vi "Configure Math.vi"(0 "VISA resource name":refnum<visa-resource-name>, 1 "Analysis Range (X) (0: Band Marker X)":u16(ring) items=["Band Marker X", "Full Range"], 5 "Measurement Type (6: Phase Noise)":u16(ring)=6 items=["AM Noise"=1, "Baseband Noise"=2, "Freq/Power"=3, "Spectrum"=4, "Transient"=5, "Phase Noise"=6, "User"=7], 7 "Select Trace (1: 1)":u16(ring)=1 items=["1"=1, "2"=2, "3"=3, "4"=4, "5"=5, "6"=6, "7"=7, "8"=8], 9 "Trace Offset (0)":dbl format="%^#_9g", 11 "error in (no error)":errorcluster, 12 "Analysis Range (Y) (0: Band Marker Y)":u16(ring) items=["Band Marker Y", "Full Range"]) -> (4 "VISA resource name out":refnum<visa-resource-name>, 15 "error out":errorcluster)   [LabVIEW 2011, in "Agilent E5052X.lvlib"]
doc: "Configures the instrument for math functions to be applied to measurements."
uses:
  Agilent E5052X.lvlib
panel:
  # "Analysis Range Settings"
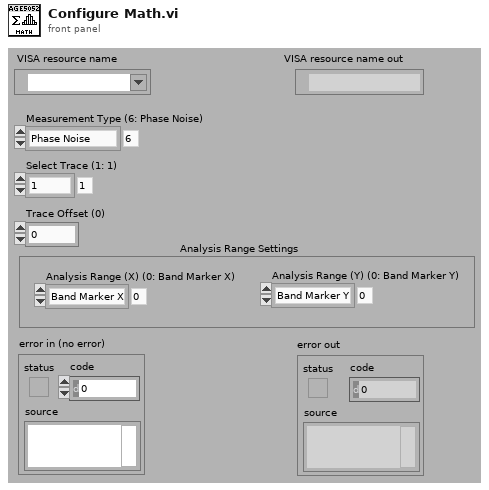
[diagram p1: front panel]
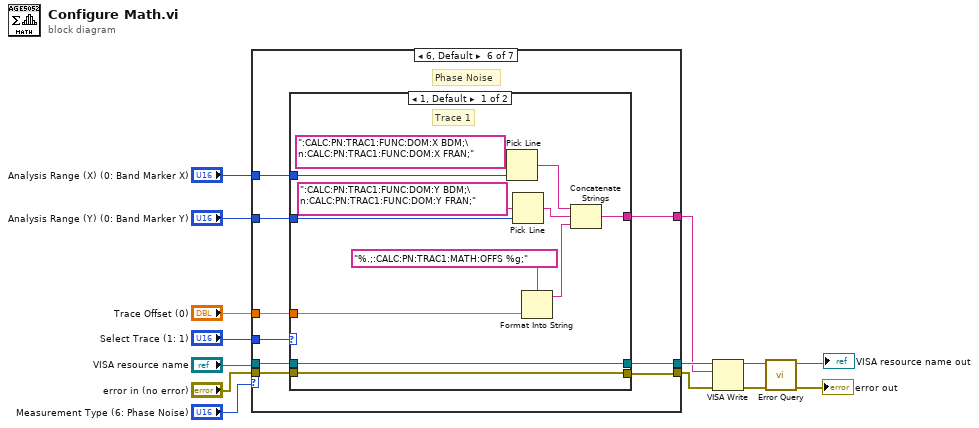
[diagram p0: block diagram]
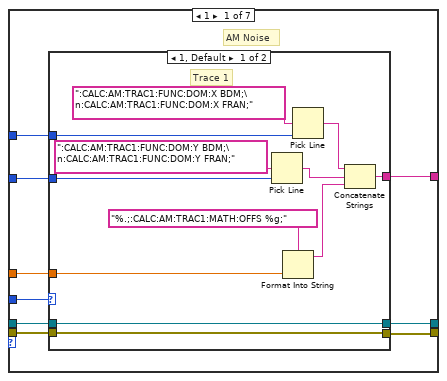
[diagram p2: hidden frame]
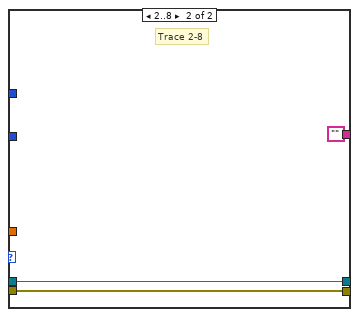
[diagram p3: hidden frame]
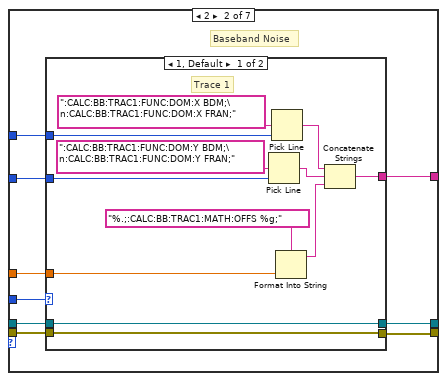
[diagram p4: hidden frame]
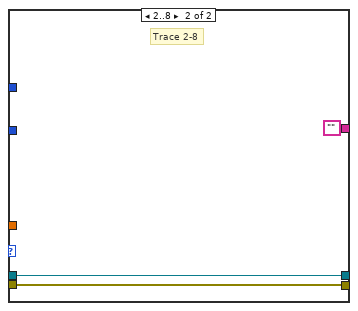
[diagram p5: hidden frame]
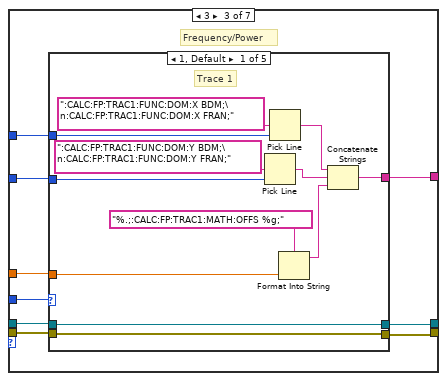
[diagram p6: hidden frame]
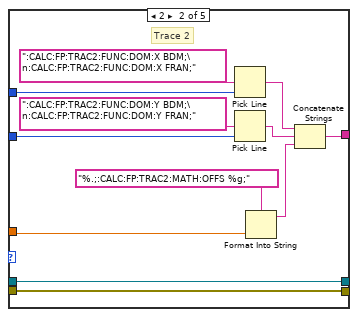
[diagram p7: hidden frame]
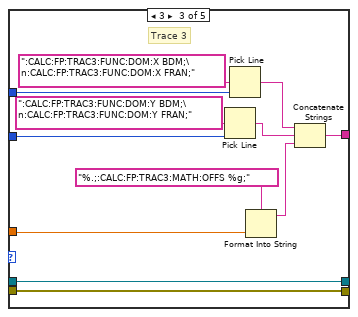
[diagram p8: hidden frame]
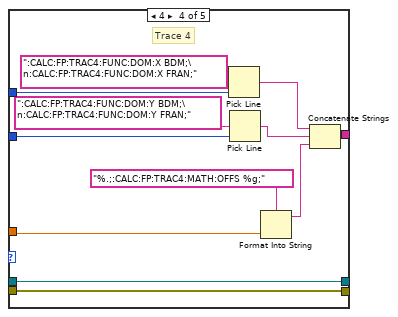
[diagram p9: hidden frame]
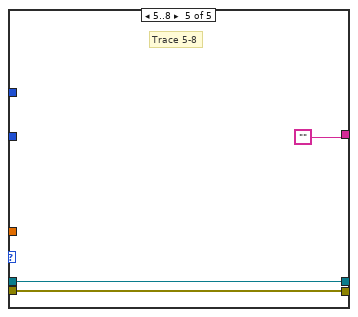
[diagram p10: hidden frame]
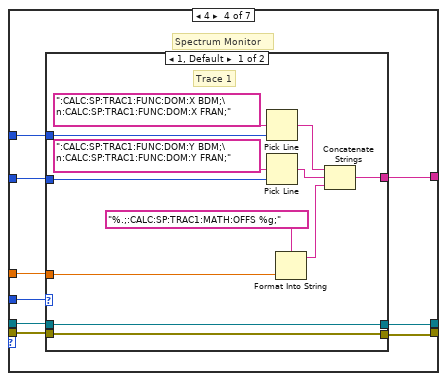
[diagram p11: hidden frame]
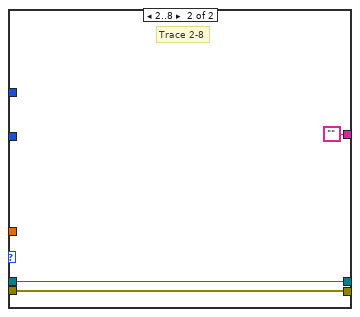
[diagram p12: hidden frame]
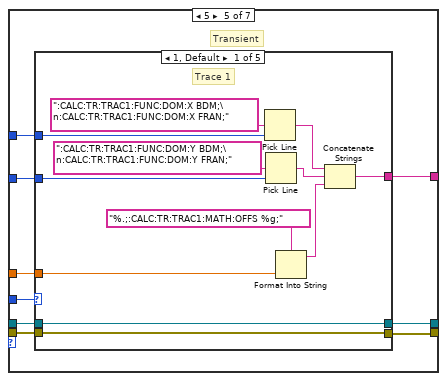
[diagram p13: hidden frame]
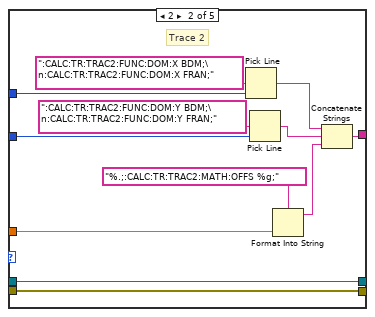
[diagram p14: hidden frame]
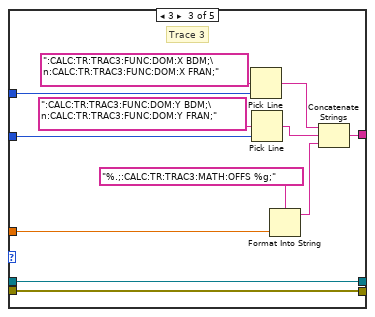
[diagram p15: hidden frame]
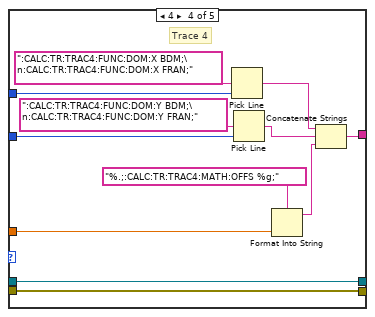
[diagram p16: hidden frame]
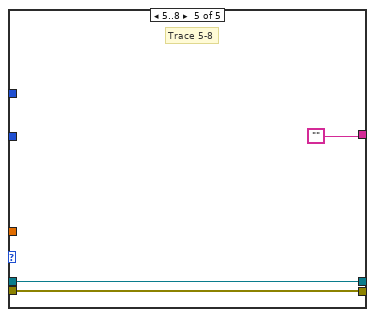
[diagram p17: hidden frame]
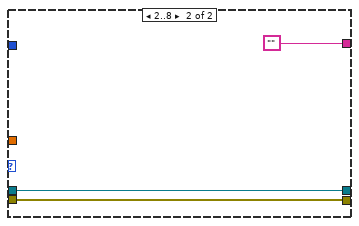
[diagram p18: hidden frame]
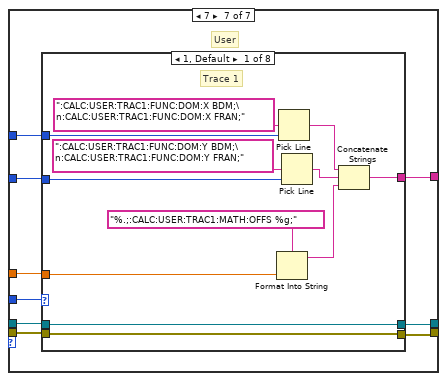
[diagram p19: hidden frame]
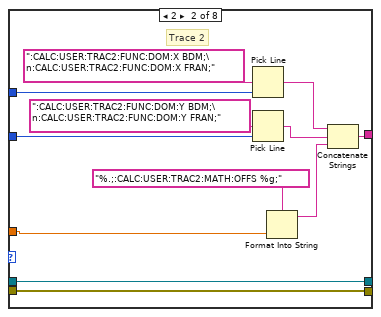
[diagram p20: hidden frame]
diagram:
  n1 = case shown="6, Default" "Measurement Type (6: Phase Noise)" {
    tunnel: "VISA resource name" -> [w23 w44 w68 w127 w151 w211 w235]
    tunnel: "error in (no error)" -> [w22 w43 w67 w126 w150 w210 w234]
    tunnel: "Select Trace (1: 1)" -> [w21 w39 w63 w128 w152 w212 w238]
    tunnel: "Trace Offset (0)" -> [w20 w45 w69 w129 w153 w213 w239]
    tunnel: "Analysis Range (Y) (0: Band Marker Y)" -> [w19 w46 w70 w130 w154 w214 w236]
    tunnel: "Analysis Range (X) (0: Band Marker X)" -> [w18 w47 w71 w131 w155 w215 w237]
    tunnel: [w17 w42 w64 w125 w149 w209 w231] -> w9
    tunnel: [w16 w41 w66 w124 w148 w208 w233] -> w11
    tunnel: [w15 w40 w65 w123 w147 w207 w232] -> w10
    frame 1 {
      # "AM Noise"
      n2 = case shown="1, Default" w21 {
        tunnel: w23 -> [w31 w38]
        tunnel: w22 -> [w30 w37]
        tunnel: w20 -> [w34 _]
        tunnel: w19 -> [w25 _]
        tunnel: w18 -> [w28 _]
        tunnel: [w32 ""] -> w17
        tunnel: [w31 w38] -> w16
        tunnel: [w30 w37] -> w15
        frame 1, Default {
          # "Trace 1"
          n3 = Pick Line(multi-line string=":CALC:AM:TRAC1:FUNC:DOM:Y BDM;\n:CALC:AM:TRAC1:FUNC:DOM:Y FRAN;", line index=w25) -> (output string=w24:string)  [unwired: 1 in]
          n4 = Format Into String(format string="%.;:CALC:AM:TRAC1:MATH:OFFS %g;", w34) -> (resulting string=w33:string)  [unwired: 2 in, 1 out]
          n5 = Pick Line(multi-line string=":CALC:AM:TRAC1:FUNC:DOM:X BDM;\n:CALC:AM:TRAC1:FUNC:DOM:X FRAN;", line index=w28) -> (output string=w27:string)  [unwired: 1 in]
          n6 = Concatenate Strings(w27, w24, w33) -> (w32:string)
        }
        frame 2..8 {
          # "Trace 2-8"
        }
      }
    }
    frame 2 {
      # "Baseband Noise"
      n7 = case shown="1, Default" w39 {
        tunnel: w44 -> [w55 w62]
        tunnel: w43 -> [w54 w61]
        tunnel: w45 -> [w58 _]
        tunnel: w46 -> [w49 _]
        tunnel: w47 -> [w52 _]
        tunnel: [w56 ""] -> w42
        tunnel: [w55 w62] -> w41
        tunnel: [w54 w61] -> w40
        frame 1, Default {
          # "Trace 1"
          n8 = Pick Line(multi-line string=":CALC:BB:TRAC1:FUNC:DOM:Y BDM;\n:CALC:BB:TRAC1:FUNC:DOM:Y FRAN;", line index=w49) -> (output string=w48:string)  [unwired: 1 in]
          n9 = Pick Line(multi-line string=":CALC:BB:TRAC1:FUNC:DOM:X BDM;\n:CALC:BB:TRAC1:FUNC:DOM:X FRAN;", line index=w52) -> (output string=w51:string)  [unwired: 1 in]
          n10 = Format Into String(format string="%.;:CALC:BB:TRAC1:MATH:OFFS %g;", w58) -> (resulting string=w57:string)  [unwired: 2 in, 1 out]
          n11 = Concatenate Strings(w51, w48, w57) -> (w56:string)
        }
        frame 2..8 {
          # "Trace 2-8"
        }
      }
    }
    frame 3 {
      # "Frequency/Power"
      n12 = case shown="1, Default" w63 {
        tunnel: w68 -> [w79 w95 w107 w119 w121]
        tunnel: w67 -> [w78 w94 w106 w118 w120]
        tunnel: w69 -> [w82 w91 w103 w115 _]
        tunnel: w70 -> [w73 w85 w97 w109 _]
        tunnel: w71 -> [w76 w88 w101 w112 _]
        tunnel: [w80 w90 w102 w114 ""] -> w64
        tunnel: [w79 w95 w107 w119 w121] -> w66
        tunnel: [w78 w94 w106 w118 w120] -> w65
        frame 1, Default {
          # "Trace 1"
          n13 = Pick Line(multi-line string=":CALC:FP:TRAC1:FUNC:DOM:Y BDM;\n:CALC:FP:TRAC1:FUNC:DOM:Y FRAN;", line index=w73) -> (output string=w72:string)  [unwired: 1 in]
          n14 = Pick Line(multi-line string=":CALC:FP:TRAC1:FUNC:DOM:X BDM;\n:CALC:FP:TRAC1:FUNC:DOM:X FRAN;", line index=w76) -> (output string=w75:string)  [unwired: 1 in]
          n15 = Format Into String(format string="%.;:CALC:FP:TRAC1:MATH:OFFS %g;", w82) -> (resulting string=w81:string)  [unwired: 2 in, 1 out]
          n16 = Concatenate Strings(w75, w72, w81) -> (w80:string)
        }
        frame 2 {
          # "Trace 2"
          n17 = Pick Line(multi-line string=":CALC:FP:TRAC2:FUNC:DOM:X BDM;\n:CALC:FP:TRAC2:FUNC:DOM:X FRAN;", line index=w88) -> (output string=w87:string)  [unwired: 1 in]
          n18 = Pick Line(multi-line string=":CALC:FP:TRAC2:FUNC:DOM:Y BDM;\n:CALC:FP:TRAC2:FUNC:DOM:Y FRAN;", line index=w85) -> (output string=w84:string)  [unwired: 1 in]
          n19 = Format Into String(format string="%.;:CALC:FP:TRAC2:MATH:OFFS %g;", w91) -> (resulting string=w92:string)  [unwired: 2 in, 1 out]
          n20 = Concatenate Strings(w87, w84, w92) -> (w90:string)
        }
        frame 3 {
          # "Trace 3"
          n21 = Pick Line(multi-line string=":CALC:FP:TRAC3:FUNC:DOM:Y BDM;\n:CALC:FP:TRAC3:FUNC:DOM:Y FRAN;", line index=w97) -> (output string=w96:string)  [unwired: 1 in]
          n22 = Pick Line(multi-line string=":CALC:FP:TRAC3:FUNC:DOM:X BDM;\n:CALC:FP:TRAC3:FUNC:DOM:X FRAN;", line index=w101) -> (output string=w100:string)  [unwired: 1 in]
          n23 = Format Into String(format string="%.;:CALC:FP:TRAC3:MATH:OFFS %g;", w103) -> (resulting string=w104:string)  [unwired: 2 in, 1 out]
          n24 = Concatenate Strings(w100, w96, w104) -> (w102:string)
        }
        frame 4 {
          # "Trace 4"
          n25 = Pick Line(multi-line string=":CALC:FP:TRAC4:FUNC:DOM:X BDM;\n:CALC:FP:TRAC4:FUNC:DOM:X FRAN;", line index=w112) -> (output string=w111:string)  [unwired: 1 in]
          n26 = Pick Line(multi-line string=":CALC:FP:TRAC4:FUNC:DOM:Y BDM;\n:CALC:FP:TRAC4:FUNC:DOM:Y FRAN;", line index=w109) -> (output string=w108:string)  [unwired: 1 in]
          n27 = Format Into String(format string="%.;:CALC:FP:TRAC4:MATH:OFFS %g;", w115) -> (resulting string=w116:string)  [unwired: 2 in, 1 out]
          n28 = Concatenate Strings(w111, w108, w116) -> (w114:string)
        }
        frame 5..8 {
          # "Trace 5-8"
        }
      }
    }
    frame 4 {
      # "Spectrum Monitor"
      n29 = case shown="1, Default" w128 {
        tunnel: w127 -> [w139 w146]
        tunnel: w126 -> [w138 w145]
        tunnel: w129 -> [w142 _]
        tunnel: w130 -> [w133 _]
        tunnel: w131 -> [w136 _]
        tunnel: [w140 ""] -> w125
        tunnel: [w139 w146] -> w124
        tunnel: [w138 w145] -> w123
        frame 1, Default {
          # "Trace 1"
          n30 = Pick Line(multi-line string=":CALC:SP:TRAC1:FUNC:DOM:X BDM;\n:CALC:SP:TRAC1:FUNC:DOM:X FRAN;", line index=w136) -> (output string=w135:string)  [unwired: 1 in]
          n31 = Pick Line(multi-line string=":CALC:SP:TRAC1:FUNC:DOM:Y BDM;\n:CALC:SP:TRAC1:FUNC:DOM:Y FRAN;", line index=w133) -> (output string=w132:string)  [unwired: 1 in]
          n32 = Format Into String(format string="%.;:CALC:SP:TRAC1:MATH:OFFS %g;", w142) -> (resulting string=w141:string)  [unwired: 2 in, 1 out]
          n33 = Concatenate Strings(w135, w132, w141) -> (w140:string)
        }
        frame 2..8 {
          # "Trace 2-8"
        }
      }
    }
    frame 5 {
      # "Transient"
      n34 = case shown="1, Default" w152 {
        tunnel: w151 -> [w163 w179 w191 w203 w205]
        tunnel: w150 -> [w162 w178 w190 w202 w204]
        tunnel: w153 -> [w166 w175 w187 w199 _]
        tunnel: w154 -> [w157 w169 w181 w194 _]
        tunnel: w155 -> [w160 w173 w184 w197 _]
        tunnel: [w164 w174 w186 w198 ""] -> w149
        tunnel: [w163 w179 w191 w203 w205] -> w148
        tunnel: [w162 w178 w190 w202 w204] -> w147
        frame 1, Default {
          # "Trace 1"
          n35 = Pick Line(multi-line string=":CALC:TR:TRAC1:FUNC:DOM:X BDM;\n:CALC:TR:TRAC1:FUNC:DOM:X FRAN;", line index=w160) -> (output string=w159:string)  [unwired: 1 in]
          n36 = Pick Line(multi-line string=":CALC:TR:TRAC1:FUNC:DOM:Y BDM;\n:CALC:TR:TRAC1:FUNC:DOM:Y FRAN;", line index=w157) -> (output string=w156:string)  [unwired: 1 in]
          n37 = Format Into String(format string="%.;:CALC:TR:TRAC1:MATH:OFFS %g;", w166) -> (resulting string=w165:string)  [unwired: 2 in, 1 out]
          n38 = Concatenate Strings(w159, w156, w165) -> (w164:string)
        }
        frame 2 {
          # "Trace 2"
          n39 = Pick Line(multi-line string=":CALC:TR:TRAC2:FUNC:DOM:X BDM;\n:CALC:TR:TRAC2:FUNC:DOM:X FRAN;", line index=w173) -> (output string=w171:string)  [unwired: 1 in]
          n40 = Pick Line(multi-line string=":CALC:TR:TRAC2:FUNC:DOM:Y BDM;\n:CALC:TR:TRAC2:FUNC:DOM:Y FRAN;", line index=w169) -> (output string=w168:string)  [unwired: 1 in]
          n41 = Format Into String(format string="%.;:CALC:TR:TRAC2:MATH:OFFS %g;", w175) -> (resulting string=w176:string)  [unwired: 2 in, 1 out]
          n42 = Concatenate Strings(w171, w168, w176) -> (w174:string)
        }
        frame 3 {
          # "Trace 3"
          n43 = Pick Line(multi-line string=":CALC:TR:TRAC3:FUNC:DOM:X BDM;\n:CALC:TR:TRAC3:FUNC:DOM:X FRAN;", line index=w184) -> (output string=w183:string)  [unwired: 1 in]
          n44 = Pick Line(multi-line string=":CALC:TR:TRAC3:FUNC:DOM:Y BDM;\n:CALC:TR:TRAC3:FUNC:DOM:Y FRAN;", line index=w181) -> (output string=w180:string)  [unwired: 1 in]
          n45 = Format Into String(format string="%.;:CALC:TR:TRAC3:MATH:OFFS %g;", w187) -> (resulting string=w188:string)  [unwired: 2 in, 1 out]
          n46 = Concatenate Strings(w183, w180, w188) -> (w186:string)
        }
        frame 4 {
          # "Trace 4"
          n47 = Pick Line(multi-line string=":CALC:TR:TRAC4:FUNC:DOM:X BDM;\n:CALC:TR:TRAC4:FUNC:DOM:X FRAN;", line index=w197) -> (output string=w196:string)  [unwired: 1 in]
          n48 = Pick Line(multi-line string=":CALC:TR:TRAC4:FUNC:DOM:Y BDM;\n:CALC:TR:TRAC4:FUNC:DOM:Y FRAN;", line index=w194) -> (output string=w192:string)  [unwired: 1 in]
          n49 = Format Into String(format string="%.;:CALC:TR:TRAC4:MATH:OFFS %g;", w199) -> (resulting string=w200:string)  [unwired: 2 in, 1 out]
          n50 = Concatenate Strings(w196, w192, w200) -> (w198:string)
        }
        frame 5..8 {
          # "Trace 5-8"
        }
      }
    }
    frame 6, Default {
      # "Phase Noise"
      n51 = case shown="1, Default" w212 {
        tunnel: w211 -> [w223 w230]
        tunnel: w210 -> [w222 w229]
        tunnel: w213 -> [w226 _]
        tunnel: w214 -> [w217 _]
        tunnel: w215 -> [w220 _]
        tunnel: [w224 ""] -> w209
        tunnel: [w223 w230] -> w208
        tunnel: [w222 w229] -> w207
        frame 1, Default {
          # "Trace 1"
          n52 = Pick Line(multi-line string=":CALC:PN:TRAC1:FUNC:DOM:X BDM;\n:CALC:PN:TRAC1:FUNC:DOM:X FRAN;", line index=w220) -> (output string=w219:string)  [unwired: 1 in]
          n53 = Pick Line(multi-line string=":CALC:PN:TRAC1:FUNC:DOM:Y BDM;\n:CALC:PN:TRAC1:FUNC:DOM:Y FRAN;", line index=w217) -> (output string=w216:string)  [unwired: 1 in]
          n54 = Format Into String(format string="%.;:CALC:PN:TRAC1:MATH:OFFS %g;", w226) -> (resulting string=w225:string)  [unwired: 2 in, 1 out]
          n55 = Concatenate Strings(w219, w216, w225) -> (w224:string)
        }
        frame 2..8 {
        }
      }
    }
    frame 7 {
      # "User"
      n56 = case shown="1, Default" w238 {
        tunnel: w235 -> [w247 w263 w275 w287 w299 w311 w323 w335]
        tunnel: w234 -> [w246 w262 w274 w286 w298 w310 w322 w334]
        tunnel: w239 -> [w250 w259 w271 w283 w295 w307 w319 w331]
        tunnel: w236 -> [w241 w253 w265 w277 w289 w301 w313 w325]
        tunnel: w237 -> [w244 w257 w269 w280 w293 w305 w316 w328]
        tunnel: [w248 w258 w270 w282 w294 w306 w318 w330] -> w231
        tunnel: [w247 w263 w275 w287 w299 w311 w323 w335] -> w233
        tunnel: [w246 w262 w274 w286 w298 w310 w322 w334] -> w232
        frame 1, Default {
          # "Trace 1"
          n57 = Format Into String(format string="%.;:CALC:USER:TRAC1:MATH:OFFS %g;", w250) -> (resulting string=w249:string)  [unwired: 2 in, 1 out]
          n58 = Pick Line(multi-line string=":CALC:USER:TRAC1:FUNC:DOM:X BDM;\n:CALC:USER:TRAC1:FUNC:DOM:X FRAN;", line index=w244) -> (output string=w243:string)  [unwired: 1 in]
          n59 = Pick Line(multi-line string=":CALC:USER:TRAC1:FUNC:DOM:Y BDM;\n:CALC:USER:TRAC1:FUNC:DOM:Y FRAN;", line index=w241) -> (output string=w240:string)  [unwired: 1 in]
          n60 = Concatenate Strings(w243, w240, w249) -> (w248:string)
        }
        frame 2 {
          # "Trace 2"
          n61 = Pick Line(multi-line string=":CALC:USER:TRAC2:FUNC:DOM:X BDM;\n:CALC:USER:TRAC2:FUNC:DOM:X FRAN;", line index=w257) -> (output string=w256:string)  [unwired: 1 in]
          n62 = Pick Line(multi-line string=":CALC:USER:TRAC2:FUNC:DOM:Y BDM;\n:CALC:USER:TRAC2:FUNC:DOM:Y FRAN;", line index=w253) -> (output string=w252:string)  [unwired: 1 in]
          n63 = Format Into String(format string="%.;:CALC:USER:TRAC2:MATH:OFFS %g;", w259) -> (resulting string=w260:string)  [unwired: 2 in, 1 out]
          n64 = Concatenate Strings(w256, w252, w260) -> (w258:string)
        }
        frame 3 {
          # "Trace 3"
          n65 = Pick Line(multi-line string=":CALC:USER:TRAC3:FUNC:DOM:Y BDM;\n:CALC:USER:TRAC3:FUNC:DOM:Y FRAN;", line index=w265) -> (output string=w264:string)  [unwired: 1 in]
          n66 = Pick Line(multi-line string=":CALC:USER:TRAC3:FUNC:DOM:X BDM;\n:CALC:USER:TRAC3:FUNC:DOM:X FRAN;", line index=w269) -> (output string=w267:string)  [unwired: 1 in]
          n67 = Format Into String(format string="%.;:CALC:USER:TRAC3:MATH:OFFS %g;", w271) -> (resulting string=w272:string)  [unwired: 2 in, 1 out]
          n68 = Concatenate Strings(w267, w264, w272) -> (w270:string)
        }
        frame 4 {
          # "Trace 4"
          n69 = Pick Line(multi-line string=":CALC:USER:TRAC4:FUNC:DOM:Y BDM;\n:CALC:USER:TRAC4:FUNC:DOM:Y FRAN;", line index=w277) -> (output string=w276:string)  [unwired: 1 in]
          n70 = Pick Line(multi-line string=":CALC:USER:TRAC4:FUNC:DOM:X BDM;\n:CALC:USER:TRAC4:FUNC:DOM:X FRAN;", line index=w280) -> (output string=w279:string)  [unwired: 1 in]
          n71 = Format Into String(format string="%.;:CALC:USER:TRAC4:MATH:OFFS %g;", w283) -> (resulting string=w284:string)  [unwired: 2 in, 1 out]
          n72 = Concatenate Strings(w279, w276, w284) -> (w282:string)
        }
        frame 5 {
          # "Trace 5"
          n73 = Pick Line(multi-line string=":CALC:USER:TRAC5:FUNC:DOM:Y BDM;\n:CALC:USER:TRAC5:FUNC:DOM:Y FRAN;", line index=w289) -> (output string=w288:string)  [unwired: 1 in]
          n74 = Pick Line(multi-line string=":CALC:USER:TRAC5:FUNC:DOM:X BDM;\n:CALC:USER:TRAC5:FUNC:DOM:X FRAN;", line index=w293) -> (output string=w291:string)  [unwired: 1 in]
          n75 = Format Into String(format string="%.;:CALC:USER:TRAC5:MATH:OFFS %g;", w295) -> (resulting string=w296:string)  [unwired: 2 in, 1 out]
          n76 = Concatenate Strings(w291, w288, w296) -> (w294:string)
        }
        frame 6 {
          # "Trace 6"
          n77 = Pick Line(multi-line string=":CALC:USER:TRAC6:FUNC:DOM:X BDM;\n:CALC:USER:TRAC6:FUNC:DOM:X FRAN;", line index=w305) -> (output string=w303:string)  [unwired: 1 in]
          n78 = Pick Line(multi-line string=":CALC:USER:TRAC6:FUNC:DOM:Y BDM;\n:CALC:USER:TRAC6:FUNC:DOM:Y FRAN;", line index=w301) -> (output string=w300:string)  [unwired: 1 in]
          n79 = Format Into String(format string="%.;:CALC:USER:TRAC6:MATH:OFFS %g;", w307) -> (resulting string=w308:string)  [unwired: 2 in, 1 out]
          n80 = Concatenate Strings(w303, w300, w308) -> (w306:string)
        }
        frame 7 {
          # "Trace 7"
          n81 = Pick Line(multi-line string=":CALC:USER:TRAC7:FUNC:DOM:Y BDM;\n:CALC:USER:TRAC7:FUNC:DOM:Y FRAN;", line index=w313) -> (output string=w312:string)  [unwired: 1 in]
          n82 = Pick Line(multi-line string=":CALC:USER:TRAC7:FUNC:DOM:X BDM;\n:CALC:USER:TRAC7:FUNC:DOM:X FRAN;", line index=w316) -> (output string=w315:string)  [unwired: 1 in]
          n83 = Format Into String(format string="%.;:CALC:USER:TRAC7:MATH:OFFS %g;", w319) -> (resulting string=w320:string)  [unwired: 2 in, 1 out]
          n84 = Concatenate Strings(w315, w312, w320) -> (w318:string)
        }
        frame 8 {
          # "Trace 8"
          n85 = Pick Line(multi-line string=":CALC:USER:TRAC8:FUNC:DOM:Y BDM;\n:CALC:USER:TRAC8:FUNC:DOM:Y FRAN;", line index=w325) -> (output string=w324:string)  [unwired: 1 in]
          n86 = Pick Line(multi-line string=":CALC:USER:TRAC8:FUNC:DOM:X BDM;\n:CALC:USER:TRAC8:FUNC:DOM:X FRAN;", line index=w328) -> (output string=w327:string)  [unwired: 1 in]
          n87 = Format Into String(format string="%.;:CALC:USER:TRAC8:MATH:OFFS %g;", w331) -> (resulting string=w332:string)  [unwired: 2 in, 1 out]
          n88 = Concatenate Strings(w327, w324, w332) -> (w330:string)
        }
      }
    }
  }
  n89 = VISA Write(VISA resource name=w11, write buffer=w9, error in (no error)=w10) -> (VISA resource name out=w8:refnum<visa-resource-name>, error out=w7:errorcluster)  [unwired: 1 out]
  n90 = call "Error Query.vi"("error in (no error)"=w7, "VISA resource name"=w8) -> ("error out"=→"error out":errorcluster, "VISA resource name out"=→"VISA resource name out":refnum<visa-resource-name>)  [unwired: 6 in, 2 out]
